vi "DelLeadingZeroes.vi"(1 "A 2":T1) -> (0 "A":T1)   [LabVIEW 2025]
uses:
  Number.ctl
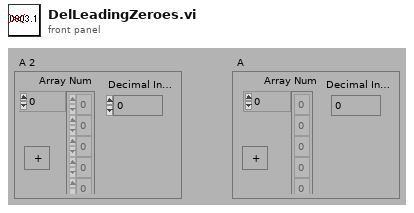
[diagram p1: front panel]
types:
  T1 = typedef "Number.ctl" = cluster{"Array Num":i8[], "Decimal Index":i32, "stop":bool}
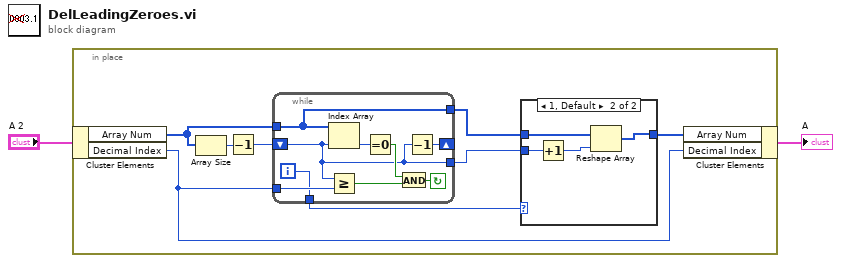
[diagram p0: block diagram]
diagram:
  n1 = in-place {
    n2 = in-place-cluster #1("A 2") -> ("Array Num"=w9:i8[], "Decimal Index"=w8:i32)
    n3 = Array Size(array=w9) -> (size(s)=w10:i32)
    n4 = Decrement(x=w10) -> (x-1=w3:i32)
    n5 = while {
      tunnel: [w21] -> w5
      tunnel: [w17] -> w7
      tunnel: w9 -> [w21]
      tunnel: w8 -> [w20]
      shift-right: [w18] -> _
      shift-left: w3 -> [w17]
      tunnel: [w16] -> w6
      i -> [w16]
      stop <- w24 continue-if-true
      n6 = Index Array(array=w21, index=w17) -> (element=w23:i8)
      n7 = Greater Or Equal?(x=w17, y=w20) -> (x >= y?=w22:bool)
      n8 = Equal To 0?(x=w23) -> (x = 0?=w19:bool)
      n9 = And(x=w19, y=w22) -> (x .and. y?=w24:bool)
      n10 = Decrement(x=w17) -> (x-1=w18:i32)
    }
    n11 = case shown="1, Default" w6 {
      tunnel: w5 -> [w11 w14]
      tunnel: [w11 w12] -> w4
      tunnel: w7 -> [_ w15]
      frame 0 {
      }
      frame 1, Default {
        n12 = Increment(x=w15) -> (x+1=w13:i32)
        n13 = Reshape Array(w14, w13) -> (w12:i8[])
      }
    }
    n14 = in-place-cluster #1("Array Num"=w4, "Decimal Index"=w8) -> (→"A":T1)
  }
